vi "Get Request Type.vi"(8 "error in (no error)":errorcluster, 11 "CreateProfile in":refnum<class "CreateProfile.lvclass">) -> (0 "error out":errorcluster, 2 "Request Type":string, 3 "CreateProfile out":refnum<class "CreateProfile.lvclass">)   [LabVIEW 2020, in "obs-websocket.lvlib" / "CreateProfile.lvclass"]
uses:
  CreateProfile.lvclass
  CreateProfile.lvclass/CreateProfile.ctl
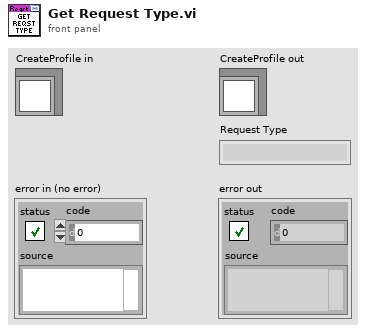
[diagram p1: front panel]
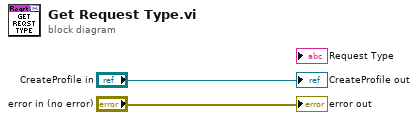
[diagram p0: block diagram]
diagram:
  "error out" <- "error in (no error)"
  "CreateProfile out" <- "CreateProfile in"
